vi "Sub_sample_unique_pin_locations.vi"(9 "Setup Parameters":T1, 10 "FEA Nodes":i32[](array[numeric]), 11 "Initial Pin Location":i32) -> (1 "Unique Samples":i32[](array[numeric]), 2 "Sample PDF":dbl[](array[numeric]), 3 "Standard Deviation":dbl)   [LabVIEW 2021]
uses:
  <vilib>/gmath/statdist.llb/Normal PDF.vi
  <vilib>/gmath/NI_Gmath.lvlib
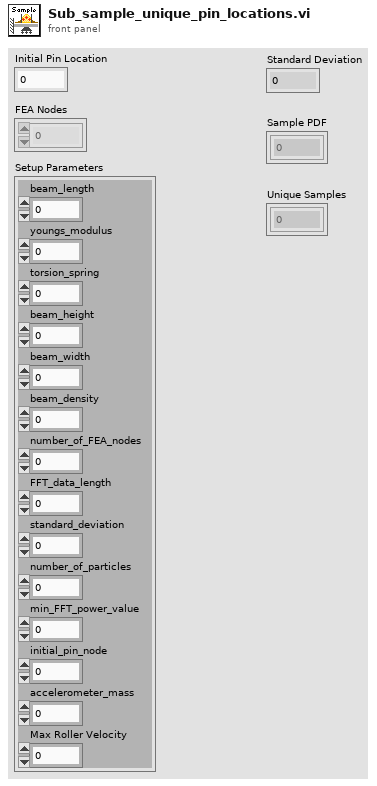
[diagram p1: front panel]
types:
  T1 = cluster{"beam_length":dbl, "youngs_modulus":dbl, "torsion_spring":dbl, "beam_height":dbl, "beam_width":dbl, "beam_density":dbl, "number_of_FEA_nodes":i32, "FFT_data_length":i32, "standard_deviation":dbl, "number_of_particles":i32, "min_FFT_power_value":dbl, "initial_pin_node":i32, "accelerometer_mass":dbl, "Max Roller Velocity":dbl}
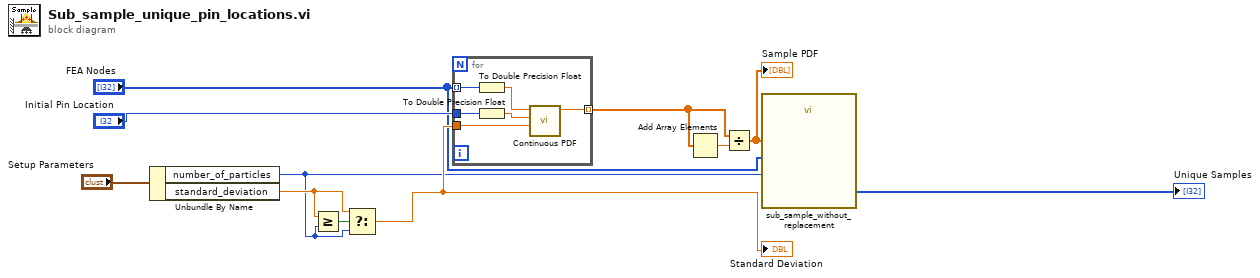
[diagram p0: block diagram]
diagram:
  n1 = Unbundle By Name("Setup Parameters") -> ("number_of_particles"=w3:i32, "standard_deviation"=w5:dbl)
  n2 = Greater Or Equal?(x=w5, y=w3) -> (x >= y?=w6:bool)
  n3 = Select(t=w5, s=w6, f=w3) -> (s? t:f=w4:dbl)
  "Standard Deviation" <- w4
  n4 = for {
    tunnel: "FEA Nodes" -> [w14] mode=indexing
    tunnel: [w17] -> w8 mode=indexing
    tunnel: "Initial Pin Location" -> [w13]
    tunnel: w4 -> [w16]
    n5 = To Double Precision Float(number=w14) -> (double precision float=w15:dbl)
    n6 = To Double Precision Float(number=w13) -> (double precision float=w12:dbl)
    n7 = call-poly <vilib>:"Continuous PDF.vi"("std"=w16, "mean"=w12, "x"=w15) -> ("pdf(x)"=w17:dbl)  [unwired: 7 in, 1 out]
  }
  n8 = Add Array Elements(numeric array=w8) -> (sum=w10:dbl)
  n9 = Divide(x=w8, y=w10) -> (x/y=w11:dbl[])
  "Sample PDF" <- w11
  n10 = call "sub_sample_without_replacement.vi"("number of unique samples"=w3, "probability"=w11, "List"="FEA Nodes") -> ("unique samples"=→"Unique Samples":i32[])  [unwired: 6 in, 2 out]
